vi "TEST.vi"() -> ()   [LabVIEW 2018, in "Config Parser SPI_3W.lvlib" / "Config Parser SPI_3W.lvclass"]
uses:
  Config Parser SPI_3W.lvclass
  Ctls/Frame Data - SPI_3W.ctl
  Ctls/RW Options.ctl
  Interfaces/File Parser Interface.lvlibp/Interfaces/File Parser Interface/File Parser Interface.lvclass
  Interfaces/File Parser Interface.lvlibp/Ctls/Protocol Type.ctl
  Interfaces/File Parser Interface.lvlibp
panel:
  out "Array":T1[](array[typedef]) {"Addr" format="%x"; "Data" format="%x"}
  out "error out":errorcluster
  in  "File Path":path
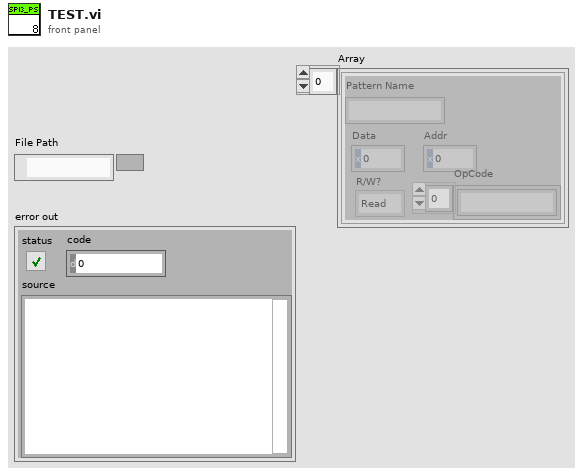
[diagram p1: front panel]
types:
  T1 = typedef "Frame Data - SPI_3W.ctl" = cluster{"Pattern Name":string, "Data":u16, "Addr":u16, "OpCode":string[], "R/W?":T2}
  T2 = typedef "RW Options.ctl" = enum16{"Read", "Write", "R/W"}
  T3 = typedef "File Parser Interface.lvlibp/Protocol Type.ctl" = enum16{"BML_LS", "BML_HS", "SPI_3W", "SPI_4W"}
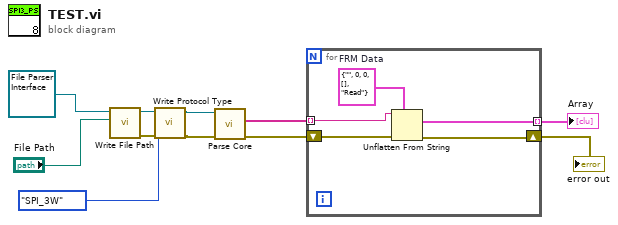
[diagram p0: block diagram]
diagram:
  n1 = call "Write File Path.vi"("File Path"="File Path", "File Parser Interface in"=refnum<class "File Parser Interface.lvclass"> refnum ("File Parser Interface.lvlibp:File Parser Interface.lvclass")) -> ("error out"=w4:errorcluster, "File Parser Interface out"=w5:refnum<class "File Parser Interface.lvclass">)  [unwired: 8 in]
  n2 = call "Write Protocol Type.vi"("error in (no error)"=w4, "Protocol Type"=Protocol_Type."SPI_3W", "File Parser Interface in"=w5) -> ("error out"=w2:errorcluster, "File Parser Interface out"=w3:refnum<class "File Parser Interface.lvclass">)  [unwired: 7 in]
  n3 = call-dynamic "Parse Core.vi"("error in (no error)"=w2, "File Parser Interface in"=w3) -> ("error out"=w10:errorcluster, "Config Array"=w11:string[])  [unwired: 7 in, 1 out]
  n4 = for {
    tunnel: w11 -> [w16] mode=indexing
    shift-right: [w14] -> w9
    shift-left: w10 -> [w15]
    tunnel: [w13] -> w8 mode=indexing
    w12 = T1 {"Pattern Name"="", "Data"=0, "Addr"=0, "OpCode"=[], "R/W?"=enum."Read"}  # FRM Data
    n5 = Unflatten From String(type=w12, binary string=w16, error in (no error)=w15) -> (value=w13:T1, error out=w14:errorcluster)  [unwired: 2 in, 1 out]
  }
  "error out" <- w9
  "Array" <- w8
